vi "edit-data.vi"(10 "Hardware Resources in":T1 {"Sample mode" items=["Hardware Timed Single Point"=12522, "Finite Samples"=10178, "Continuous Samples"=10123]}, 11 "data":waveform(dbl)[](array[waveform])) -> (3 "Array of Waveform":waveform(dbl)[](array[waveform]))   [LabVIEW 2018, in "Acquisition.lvlib"]
uses:
  Acquisition.lvlib
  Hardware Configuration.ctl
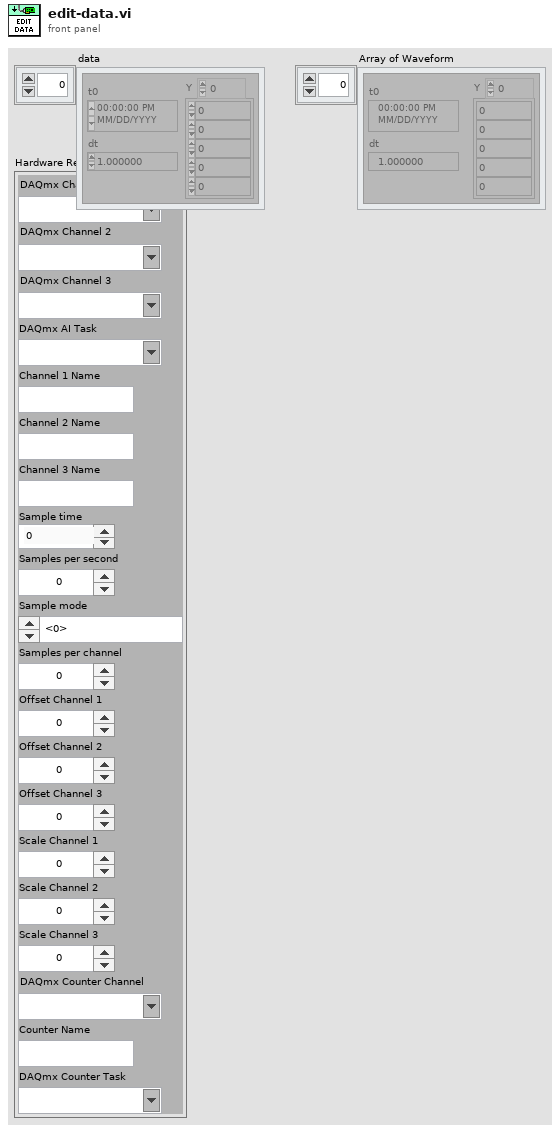
[diagram p1: front panel]
types:
  T1 = typedef "Acquisition.lvlib/Hardware Configuration.ctl" = cluster{"DAQmx Channel 1":tag, "DAQmx Channel 2":tag, "DAQmx Channel 3":tag, "DAQmx AI Task":refnum<k21>, "Channel 1 Name":string, "Channel 2 Name":string, "Channel 3 Name":string, "Sample time":u32, "Samples per second":dbl, "Sample mode":u16, "Samples per channel":i32, "Offset Channel 1":dbl, "Offset Channel 2":dbl, "Offset Channel 3":dbl, "Scale Channel 1":dbl, "Scale Channel 2":dbl, "Scale Channel 3":dbl, "DAQmx Counter Channel":tag, "Counter Name":string, "DAQmx Counter Task":refnum<k21>}
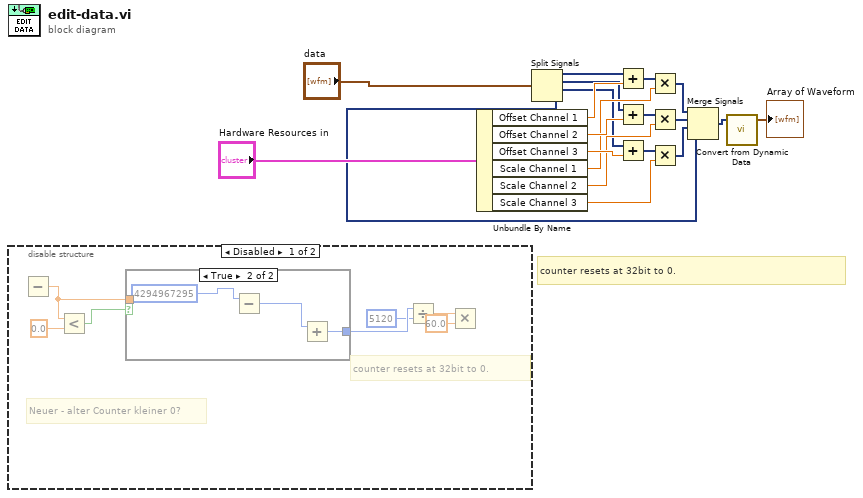
[diagram p0: block diagram]
diagram:
  # "counter resets at 32bit to 0."
  n1 = disable-structure shown="Disabled" {
    frame Disabled {
      # "Neuer - alter Counter kleiner 0?"
      # "counter resets at 32bit to 0."
      n2 = Subtract() -> (x-y=w21:dbl)  [unwired: 2 in]
      n3 = Less?(x=w21, y=0.0) -> (x < y?=w23:bool)
      n4 = case shown="True" w23 {
        tunnel: [_ w28] -> w27
        tunnel: w21 -> [_ _]
        frame False {
        }
        frame True {
          n5 = Subtract(x=u32 4294967295 ("y")) -> (x-y=w29:u32)  [unwired: 1 in]
          n6 = Add(x=w29) -> (x+y=w28:u32)  [unwired: 1 in]
        }
      }
      n7 = Divide(x=w27, y=u32 5120) -> (x/y=w25:dbl)
      n8 = Multiply(x=w25, y=60.0) -> ()  [unwired: 1 out]
    }
    frame Enabled {
    }
  }
  n9 = Unbundle By Name("Hardware Resources in") -> ("Offset Channel 1"=w15:dbl, "Offset Channel 2"=w17:dbl, "Offset Channel 3"=w19:dbl, "Scale Channel 1"=w16:dbl, "Scale Channel 2"=w18:dbl, "Scale Channel 3"=w20:dbl)
  n10 = Split Signals("data") -> (w3:dynamicdata, w4:dynamicdata, w5:dynamicdata, w1:dynamicdata)  [unwired: 4 in]
  n11 = Add(x=w3, y=w15) -> (x+y=w6:dynamicdata)
  n12 = Add(x=w4, y=w17) -> (x+y=w7:dynamicdata)
  n13 = Add(x=w5, y=w19) -> (x+y=w8:dynamicdata)
  n14 = Multiply(x=w6, y=w16) -> (x*y=w9:dynamicdata)
  n15 = Multiply(x=w7, y=w18) -> (x*y=w10:dynamicdata)
  n16 = Multiply(x=w8, y=w20) -> (x*y=w11:dynamicdata)
  n17 = Merge Signals(w9, w10, w11, w1) -> (w12:dynamicdata)
  n18 = call "Convert from Dynamic Data"("Dynamic Data Type"=w12) -> ("Array of Waveform"=→"Array of Waveform":waveform(dbl)[])  [unwired: 3 in]
